vi "PathExt.vi"(1 "New Extension":string, 2 "Down Load File Path":path) -> (0 "Down Load Log File Path":path)   [LabVIEW 2020]
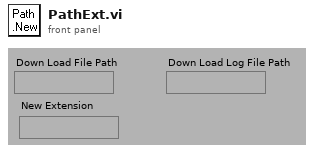
[diagram p1: front panel]
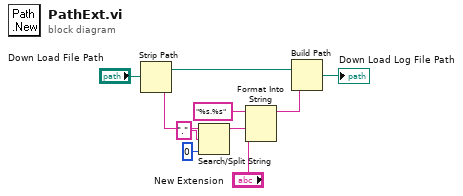
[diagram p0: block diagram]
diagram:
  n1 = Strip Path(path="Down Load File Path") -> (stripped path=w8:path, name=w9:string)
  n2 = Search/Split String(string=w9, search string/char (-)=".", offset (0)=0) -> (substring before match=w6:string)  [unwired: 2 out]
  n3 = Format Into String(format string="%s.%s", w6, "New Extension") -> (resulting string=w7:string)  [unwired: 2 in, 1 out]
  n4 = Build Path(base path=w8, name or relative path=w7) -> (appended path=→"Down Load Log File Path":path)
